vi "setup.vi"() -> (0 "error 2":errorcluster caption="error", 3 "error":errorcluster)   [LabVIEW 2017]
uses:
  Lib_code.lvlib
panel:
  out "error 3":errorcluster caption="error out 2"
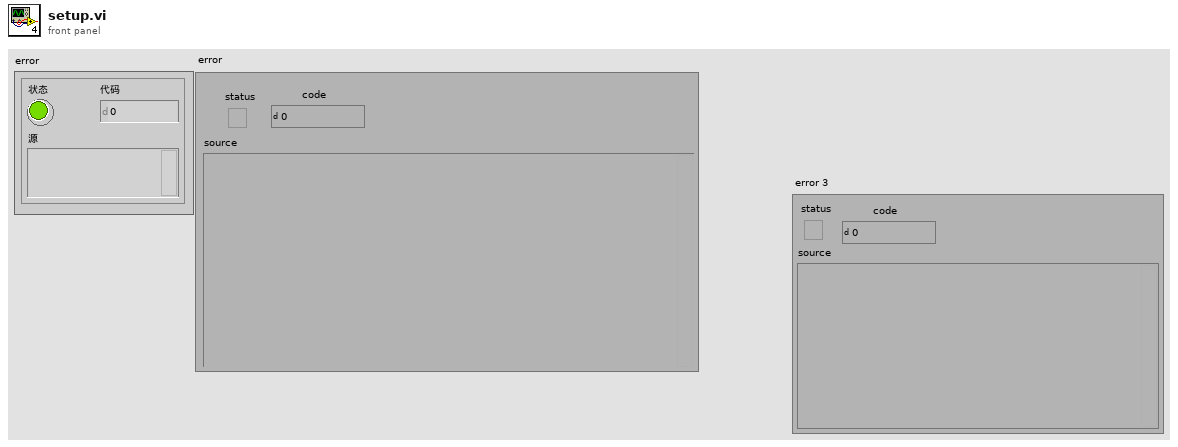
[diagram p1: front panel]
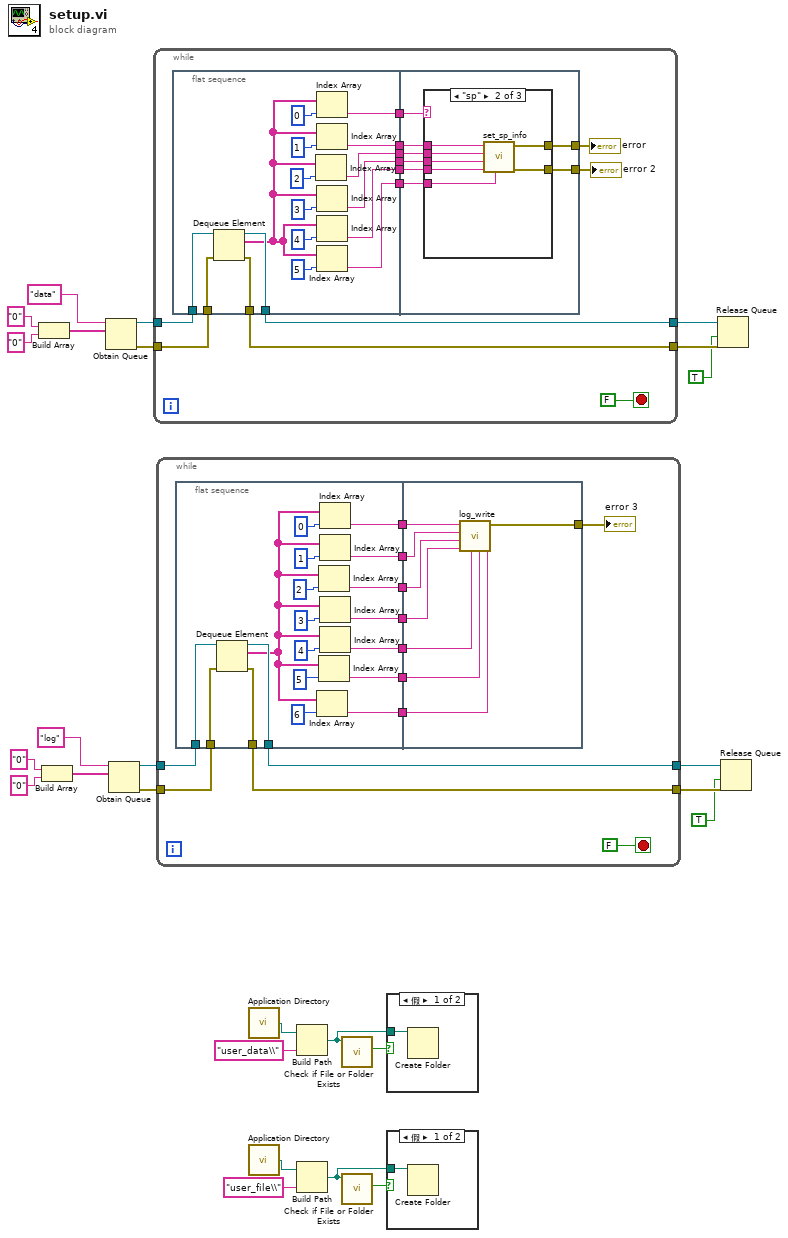
[diagram p0: block diagram]
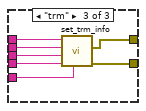
[diagram p5: hidden frame]
diagram:
  n1 = Build Array("0" ("元素"), "0" ("元素")) -> (w23:string[])
  n2 = Build Array("0" ("元素"), "0" ("元素")) -> (w14:string[])
  n3 = Obtain Queue(name (unnamed)="data" ("名称（未命名）"), element data type=w23) -> (queue out=w19:refnum<queue>, error out=w18:errorcluster)  [unwired: 3 in, 1 out]
  n4 = Obtain Queue(name (unnamed)="log" ("名称（未命名）"), element data type=w14) -> (queue out=w10:refnum<queue>, error out=w9:errorcluster)  [unwired: 3 in, 1 out]
  n5 = while {
    tunnel: w18 -> [w36]
    tunnel: [w38] -> w21
    tunnel: w19 -> [w37]
    tunnel: [w39] -> w22
    stop <- FALSE stop-if-true
    n6 = flat-sequence {
      tunnel: [w56] -> w39
      tunnel: [w55] -> w38
      tunnel: w37 -> [w54]
      tunnel: w36 -> [w53]
      tunnel: [w40] -> w34
      tunnel: [w46] -> w33
      tunnel: [w45] -> w32
      tunnel: [w44] -> w31
      tunnel: [w42] -> w30
      tunnel: [w41] -> w29
      tunnel: w34 -> [w64]
      tunnel: w33 -> [w63]
      tunnel: w32 -> [w62]
      tunnel: w31 -> [w61]
      tunnel: w30 -> [w60]
      tunnel: w29 -> [w59]
      tunnel: [w58] -> w27
      tunnel: [w57] -> w28
      frame #0 {
        n7 = Dequeue Element(queue=w54, error in (no error)=w53) -> (queue out=w56:refnum<queue>, element=w43:string[], error out=w55:errorcluster)  [unwired: 1 in, 1 out]
        n8 = Index Array(array=w43, index=2 ("索引")) -> (element=w45:string)
        n9 = Index Array(array=w43, index=0 ("索引")) -> (element=w40:string)
        n10 = Index Array(array=w43, index=1 ("索引")) -> (element=w46:string)
        n11 = Index Array(array=w43, index=3 ("索引")) -> (element=w44:string)
        n12 = Index Array(array=w43, index=4 ("索引")) -> (element=w42:string)
        n13 = Index Array(array=w43, index=5 ("索引")) -> (element=w41:string)
      }
      frame #1 {
        n14 = case shown="\"sp\"" w64 {
          tunnel: w63 -> [_ w71 w76]
          tunnel: w62 -> [_ w70 w75]
          tunnel: w61 -> [_ w69 w74]
          tunnel: w60 -> [_ w68 w73]
          tunnel: w59 -> [_ w67 w72]
          tunnel: [_ w66 w78] -> w58
          tunnel: [_ w65 w77] -> w57
          frame "假", Default {
          }
          frame "sp" {
            n15 = call "set_sp_info.vi"("yw"=w67, "sp_shuoming"=w68, "sp_yijian"=w69, "id"=w70, "lc_num"=w71) -> ("error 2"=w65:errorcluster, "error"=w66:errorcluster)  [unwired: 5 in]
          }
          frame "trm" {
            n16 = call "set_trm_info.vi"("yw"=w72, "sp_shuoming"=w73, "sp_yijian"=w74, "id"=w75, "lc_num"=w76) -> ("error"=w77:errorcluster, "error 2"=w78:errorcluster)  [unwired: 5 in]
          }
        }
      }
    }
    "error" <- w27
    "error 2" <- w28
  }
  n17 = while {
    tunnel: w9 -> [w88]
    tunnel: [w90] -> w12
    tunnel: w10 -> [w89]
    tunnel: [w91] -> w13
    stop <- FALSE stop-if-true
    n18 = flat-sequence {
      tunnel: [w110] -> w91
      tunnel: [w109] -> w90
      tunnel: w89 -> [w108]
      tunnel: w88 -> [w107]
      tunnel: [w97] -> w86
      tunnel: [w101] -> w85
      tunnel: [w100] -> w84
      tunnel: [w99] -> w83
      tunnel: [w98] -> w82
      tunnel: [w95] -> w80
      tunnel: [w92] -> w79
      tunnel: w86 -> [w118]
      tunnel: w85 -> [w117]
      tunnel: w84 -> [w116]
      tunnel: w83 -> [w115]
      tunnel: w82 -> [w114]
      tunnel: [w112] -> w81
      tunnel: w80 -> [w113]
      tunnel: w79 -> [w111]
      frame #0 {
        n19 = Dequeue Element(queue=w108, error in (no error)=w107) -> (queue out=w110:refnum<queue>, element=w93:string[], error out=w109:errorcluster)  [unwired: 1 in, 1 out]
        n20 = Index Array(array=w93, index=6 ("索引")) -> (element=w92:string)
        n21 = Index Array(array=w93, index=2 ("索引")) -> (element=w100:string)
        n22 = Index Array(array=w93, index=5 ("索引")) -> (element=w95:string)
        n23 = Index Array(array=w93, index=0 ("索引")) -> (element=w97:string)
        n24 = Index Array(array=w93, index=1 ("索引")) -> (element=w101:string)
        n25 = Index Array(array=w93, index=3 ("索引")) -> (element=w99:string)
        n26 = Index Array(array=w93, index=4 ("索引")) -> (element=w98:string)
      }
      frame #1 {
        n27 = call "log_write.vi"("type"=w111, "neirong"=w113, "ip_add"=w114, "datetime"=w115, "action"=w116, "yw"=w117, "user"=w118) -> ("error"=w112:errorcluster)  [unwired: 4 in]
      }
    }
    "error 3" <- w81
  }
  n28 = call <vilib>:"Application Directory.vi"() -> ("Application Directory"=w8:path)
  n29 = call <vilib>:"Application Directory.vi"() -> ("Application Directory"=w4:path)
  n30 = Build Path(base path=w8, name or relative path="user_data\\" ("字符串")) -> (appended path=w5:path)
  n31 = Build Path(base path=w4, name or relative path="user_file\\" ("字符串")) -> (appended path=w1:path)
  n32 = call <vilib>:"Check if File or Folder Exists.vi"("path"=w5) -> ("file or folder exists?"=w6:bool)  [unwired: 8 in, 2 out]
  n33 = call <vilib>:"Check if File or Folder Exists.vi"("path"=w1) -> ("file or folder exists?"=w2:bool)  [unwired: 8 in, 2 out]
  n34 = case shown="假" w6 {
    tunnel: w5 -> [w119 _]
    frame False {
      n35 = Create Folder(path (use dialog)=w119) -> ()  [unwired: 2 in, 3 out]
    }
    frame True {
    }
  }
  n36 = case shown="假" w2 {
    tunnel: w1 -> [w120 _]
    frame False {
      n37 = Create Folder(path (use dialog)=w120) -> ()  [unwired: 2 in, 3 out]
    }
    frame True {
    }
  }
  n38 = Release Queue(queue=w22, force destroy? (F)=TRUE ("强制销毁？(F)"), error in (no error)=w21) -> ()  [unwired: 3 out]
  n39 = Release Queue(queue=w13, force destroy? (F)=TRUE ("强制销毁？(F)"), error in (no error)=w12) -> ()  [unwired: 3 out]
